vi "SetPowerDissipatedFactor.vi"(8 "error in (no error)":errorcluster, 9 "Value":dbl format="%#_13g", 10 "Label":string, 11 "Laser in":refnum<class "Laser.lvclass">) -> (0 "error out":errorcluster, 3 "Laser out":refnum<class "Laser.lvclass">)   [LabVIEW 2020, in "Laser.lvlib" / "Laser.lvclass"]
uses:
  Laser.lvclass
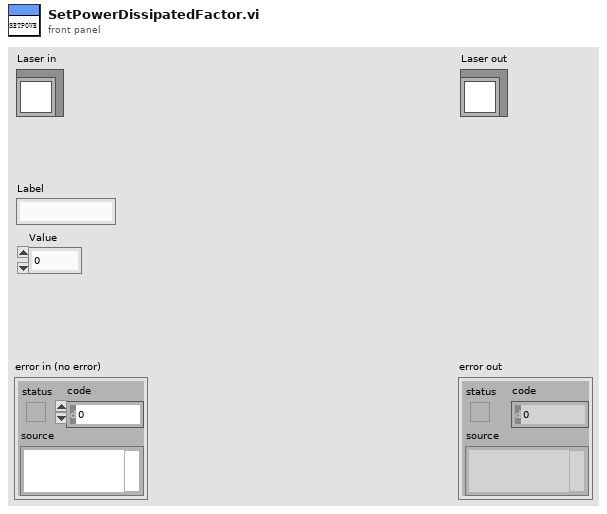
[diagram p1: front panel]
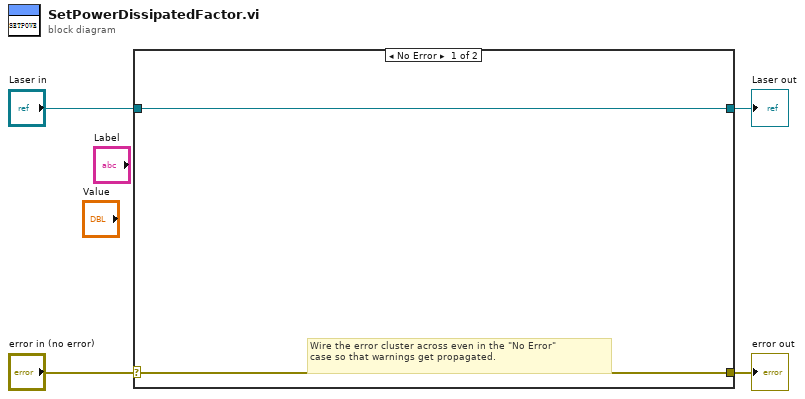
[diagram p0: block diagram]
diagram:
  n1 = case shown="No Error" "error in (no error)" {
    selector: "error in (no error)" -> [w5 w8]
    tunnel: [w5 w8] -> w3
    tunnel: [w6 w7] -> w1
    tunnel: "Laser in" -> [w6 w7]
    frame No Error {
      # "Wire the error cluster across even in the \"No Error\"\ncase so that warnings get propagated."
    }
    frame Error {
    }
  }
  "error out" <- w3
  "Laser out" <- w1
